vi "Ic_Image_Rotation.vi"(8 "error in (no error)":errorcluster, 10 "degree":dbl, 11 "2D array in":u8[][](array[numeric])) -> (0 "error out":errorcluster, 3 "2D array out":u8[][](array[numeric]))   [LabVIEW 2013]
uses:
  SLM_Control_VI_source/Image_Control.dll
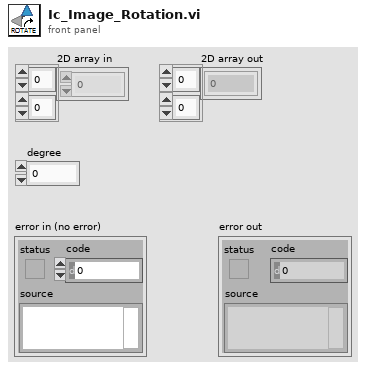
[diagram p1: front panel]
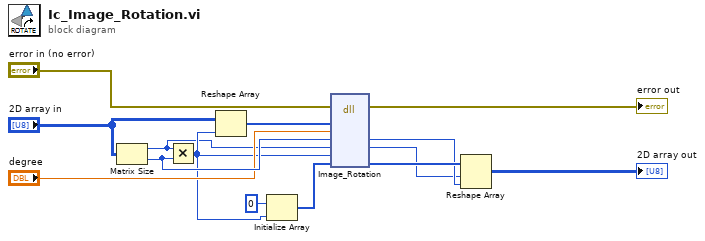
[diagram p0: block diagram]
diagram:
  n1 = Matrix Size(0:"2D array in") -> (1:w1:i32, 2:w13:i32)
  n2 = Multiply(x=w1, y=w13) -> (x*y=w3:i32)
  n3 = Reshape Array("2D array in", w3) -> (w12:u8[])
  n4 = Initialize Array(u8 0 ("要素"), w3) -> (w2:u8[])
  n5 = dll-call lib="C:/Users/hs5921/Desktop/SLM_Control_VI_source/Image_Control.dll" fn="Image_Rotation"(error in="error in (no error)", "1DArrayIn"=w12, "degree"="degree", "X_pixel_target"=w13, "Y_pixel_target"=w1, "targetDataSize"=w3, "1DArrayOut"=w2) -> (error out=→"error out":errorcluster, "X_pixel_target"=w10:i32, "Y_pixel_target"=w9:i32, "1DArrayOut"=w11:u8[])  [unwired: 6 in, 1 out]
  n6 = Reshape Array(w11, w9, w10) -> (→"2D array out":u8[][])
